vi "gpstoservo.vi"(2 "GPS Input":T3, 3 "Servo In Cluster":T2) -> (1 "Servo Out Cluster":T1)   [LabVIEW 2014]
uses:
  <vilib>/imath/engines/lvmath2/RunTimeEngine/Managers/WorkSpace/UID Generator.vi
  <vilib>/imath/engines/lvmath2/RunTimeEngine/RunTimeType/NIMS_RunTimeType_From StrictType (excl LVString).vi
  <instcachedir>/0/NIMS_RunTimeType_From StrictType (excl LVString)_15A5391EEA9C4AACB9955AC755B83D29.lvgen/NIMS_RunTimeType_From StrictType (excl LVString)_15A5391EEA9C4AACB9955AC755B83D29_000.vi
  <vilib>/imath/engines/lvmath2/RunTimeEngine/LocalVariableDefStatement/MC_LocalVariableDefStatement_Display.vi
  <vilib>/imath/engines/lvmath2/RunTimeEngine/ArithmeticOperatorToken/NIMS_ArithmeticOperator_power(S).vi
  <instcachedir>/0/NIMS_ArithmeticOperator_power(S)_CAFE680B12A64A3A8F5E28A20C679B7D.lvgen/NIMS_ArithmeticOperator_power(S)_CAFE680B12A64A3A8F5E28A20C679B7D_010.vi
  <vilib>/imath/engines/lvmath2/RunTimeEngine/BuiltInFunctions/atan/NIMS_atan(C).vi
  <instcachedir>/0/NIMS_atan(C)_ADA0F71768B44E988561745E09F50C74.lvgen/NIMS_atan(C)_ADA0F71768B44E988561745E09F50C74_001.vi
  <instcachedir>/0/NIMS_ArithmeticOperator_power(S)_CAFE680B12A64A3A8F5E28A20C679B7D.lvgen/NIMS_ArithmeticOperator_power(S)_CAFE680B12A64A3A8F5E28A20C679B7D_009.vi
  <vilib>/imath/engines/lvmath2/RunTimeEngine/ErrorHandling/NIMS_Create Error From Enums.vi
  <vilib>/imath/engines/lvmath2/RunTimeEngine/Managers/SymbolTable/Clear UID.vi
  <vilib>/imath/engines/lvmath2/RunTimeEngine/NodeEndStatement/NIMS_NodeEndStatement_Output.vi
  <instcachedir>/0/NIMS_NodeEndStatement_Output_53EC0D466D134D7ABD903AC30B43404B.lvgen/NIMS_NodeEndStatement_Output_53EC0D466D134D7ABD903AC30B43404B_001.vi
  <vilib>/imath/engines/lvmath2/RunTimeEngine/ErrorHandling/NIMS_Finalize Error.vi
  <vilib>/gmath/NI_Gmath.lvlib
  <vilib>/imath/engines/lvmath2/RunTimeEngine/Managers/SymbolTable/NIMS_WorkSpace.lvlib
panel:
  out "Calculated Servo Angles":cluster{"gamma  (x)":dbl, "theta (y)":dbl}
  in  "R (radius of roation of the Y-axis)":dbl
  in  "L (to board from servo)":dbl
  # "Configurable Parameters"
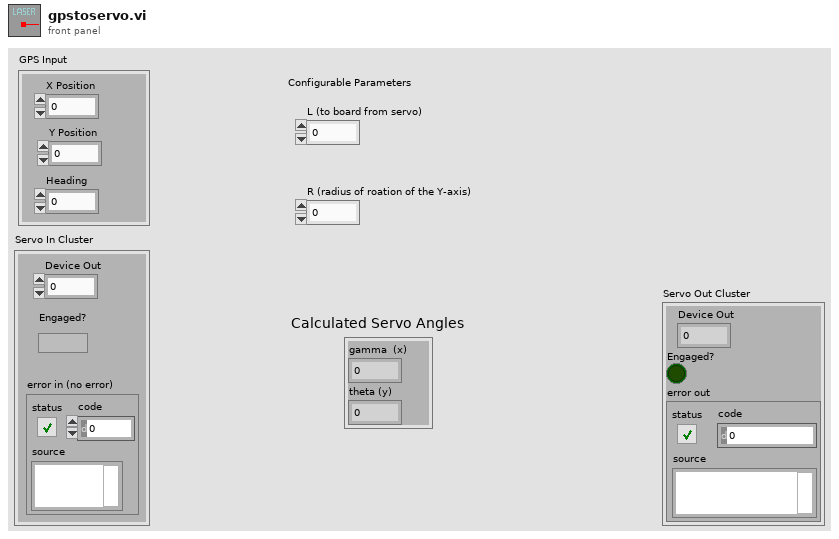
[diagram p1: front panel]
types:
  T1 = cluster{"Device Out":i32, "Engaged?":bool, "error out":errorcluster}
  T2 = cluster{"Device Out":i32, "Engaged?":bool, "error in (no error)":errorcluster}
  T3 = cluster{"X Position":i32, "Y Position":i32, "Heading":dbl}
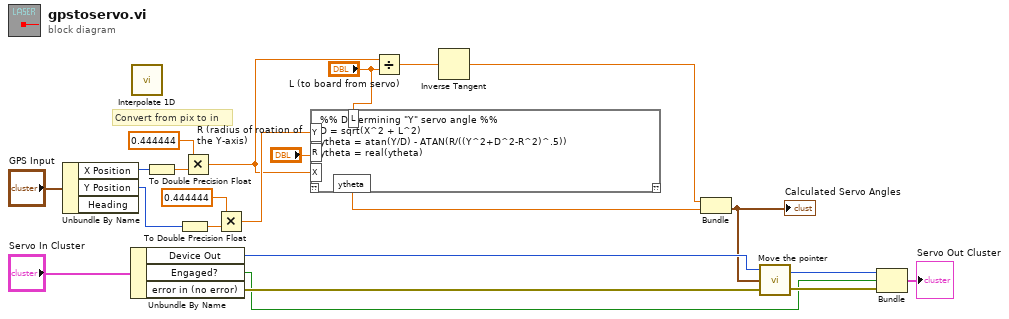
[diagram p0: block diagram]
diagram:
  # "Convert from pix to in"
  n1 = Unbundle By Name("GPS Input") -> ("X Position"=w11:i32, "Y Position"=w6:i32)  [unwired: 1 out]
  n2 = Unbundle By Name("Servo In Cluster") -> ("Device Out"=w19:i32, "Engaged?"=w13:bool, "error in (no error)"=w20:errorcluster)
  n3 = call <vilib>:"Interpolate 1D.vi"() -> ()  [unwired: 9 in, 3 out]
  n4 = To Double Precision Float(number=w11) -> (double precision float=w10:dbl)
  n5 = To Double Precision Float(number=w6) -> (double precision float=w8:dbl)
  n6 = Multiply(x=0.444444, y=w10) -> (x*y=w4:dbl)
  n7 = Multiply(x=0.444444, y=w8) -> (x*y=w5:dbl)
  n8 = mathscript code="%% Determining \"Y\" servo angle %%\nD = sqrt(X^2 + L^2)\nytheta = atan(Y/D) - ATAN(R/((Y^2+D^2-R^2)^.5))\nytheta = real(ytheta)"("Y"=w5, "X"=w4, "R"="R (radius of roation of the Y-axis)", "L"="L (to board from servo)") -> ("ytheta"=w1:dbl)  [unwired: 1 in, 1 out]
  n9 = Divide(x=w4, y="L (to board from servo)") -> (x/y=w17:dbl)
  n10 = Inverse Tangent(1:w17) -> (0:w2:dbl)
  n11 = Bundle(w2, "ytheta"=w1) -> (w18:cluster{dbl, "ytheta":dbl})  [unwired: 1 in]
  "Calculated Servo Angles" <- w18
  n12 = call "Move the pointer.vi"("error in (no error)"=w20, "Servo Angles"=w18, "Device In"=w19) -> ("error out"=w15:errorcluster, "Device Out"=w14:i32)
  n13 = Bundle("Device Out"=w14, "Engaged?"=w13, "error out"=w15) -> (→"Servo Out Cluster":T1)  [unwired: 1 in]
